vi "Reset Eload.vi"(8 "error in":errorcluster, 11 "Electronic Load in":refnum<class "Electronic Load.lvclass">) -> (0 "error out":errorcluster, 3 "Electronic Load out":refnum<class "Electronic Load.lvclass">)   [LabVIEW 2019, in "Electronic Load.lvlib" / "Electronic Load.lvclass"]
uses:
  Library/Electronic Load.lvclass
  C:/Users/Public/Documents/Development/builds/Engine/Monitored Actor.lvlibp/Monitored Actor/Monitored Actor/Monitored Actor.lvclass
  C:/Users/Public/Documents/Development/builds/Instruments/Instruments.lvlibp/Library/Instruments.lvclass
  Library/Electronic Load.lvclass/Electronic Load.ctl
  Custom Controls/E-Load Function.ctl
  Custom Controls/E-Load Mode.ctl
  Custom Controls/OCP Settings.ctl
  builds/Engine/Monitored Actor.lvlibp/Monitored Actor/Monitored Actor/Read Actor Label.vi
  builds/Instruments/Instruments.lvlibp/Private/Polymorphic/Special/Event from String.vi
  builds/Instruments/Instruments.lvlibp/Accessors/Command with Logging.vi
  builds/Instruments/Instruments.lvlibp/Library/Instruments.lvclass
  builds/Instruments/Instruments.lvlibp
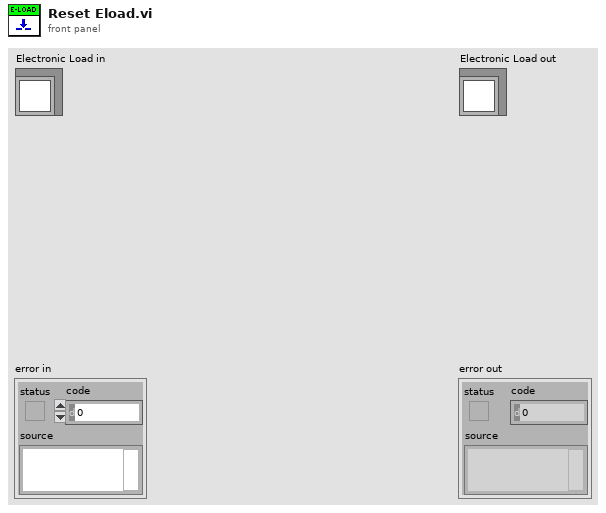
[diagram p1: front panel]
types:
  T1 = typedef "Electronic Load.lvlib/Electronic Load.lvclass/OCP Settings.ctl" = cluster{"OCP_Enabled":bool, "OCP Level":dbl, "OCP Delay":dbl}
  T2 = typedef "Electronic Load.lvlib/Electronic Load.lvclass/E-Load Function.ctl" = cluster{"Mode":T3, "Input Level":dbl, "Output":bool, "Slew Rate":dbl}
  T3 = typedef "Electronic Load.lvlib/Electronic Load.lvclass/E-Load Mode.ctl" = enum16{"Current", "Resistance", "Voltage"}
  T4 = cluster{"Timestamp":timestamp, "Description":string, "Data":string}
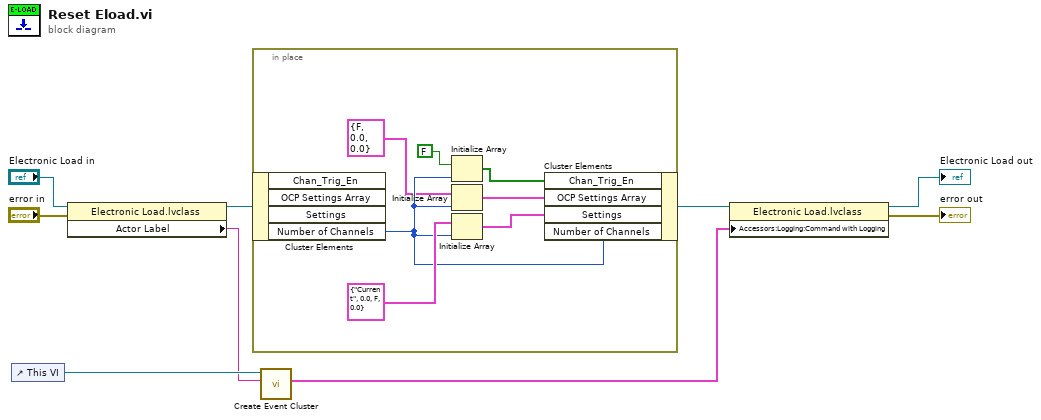
[diagram p0: block diagram]
diagram:
  n1 = control-ref of="This VI"() -> (w7:refnum<vi>)
  n2 = property class="Electronic Load.lvclass"(reference="Electronic Load in", error in="error in") -> (reference out=w3:refnum<class "Electronic Load.lvclass">, "Actor Label"=w6:string)  [unwired: 1 out]
  n3 = in-place {
    n4 = in-place-cluster #1(w3) -> ("Number of Channels"=w14:i32)  [unwired: 3 out]
    n5 = Initialize Array(FALSE, w14) -> (w10:bool[])
    n6 = Initialize Array(T1 {"OCP_Enabled"=FALSE, "OCP Level"=0.0, "OCP Delay"=0.0} ("OCP Settings"), w14) -> (w12:T1[])
    n7 = Initialize Array(T2 {"Mode"=enum."Current", "Input Level"=0.0, "Output"=FALSE, "Slew Rate"=0.0} ("Function"), w14) -> (w15:T2[])
    n8 = in-place-cluster #1("Chan_Trig_En"=w10, "OCP Settings Array"=w12, "Settings"=w15, "Number of Channels"=w14) -> (w2:refnum<class "Electronic Load.lvclass">)
  }
  n9 = call-poly "Create Event Cluster.vi"("Value"=w6, "VI Refnum"=w7) -> ("Event Data"=w1:T4)  [unwired: 9 in]
  n10 = property class="Electronic Load.lvclass"(reference=w2, "Accessors:Logging:Command with Logging"=w1) -> (reference out=→"Electronic Load out":refnum<class "Electronic Load.lvclass">, error out=→"error out":errorcluster)  [unwired: 1 in]
